vi "FTW-JSON-Interpret-Path.vi"(1 "JSON String":string) -> (0 "LabVIEW Path":path)   [LabVIEW 2015]
panel:
  # "Inputs"
  # "Outputs"
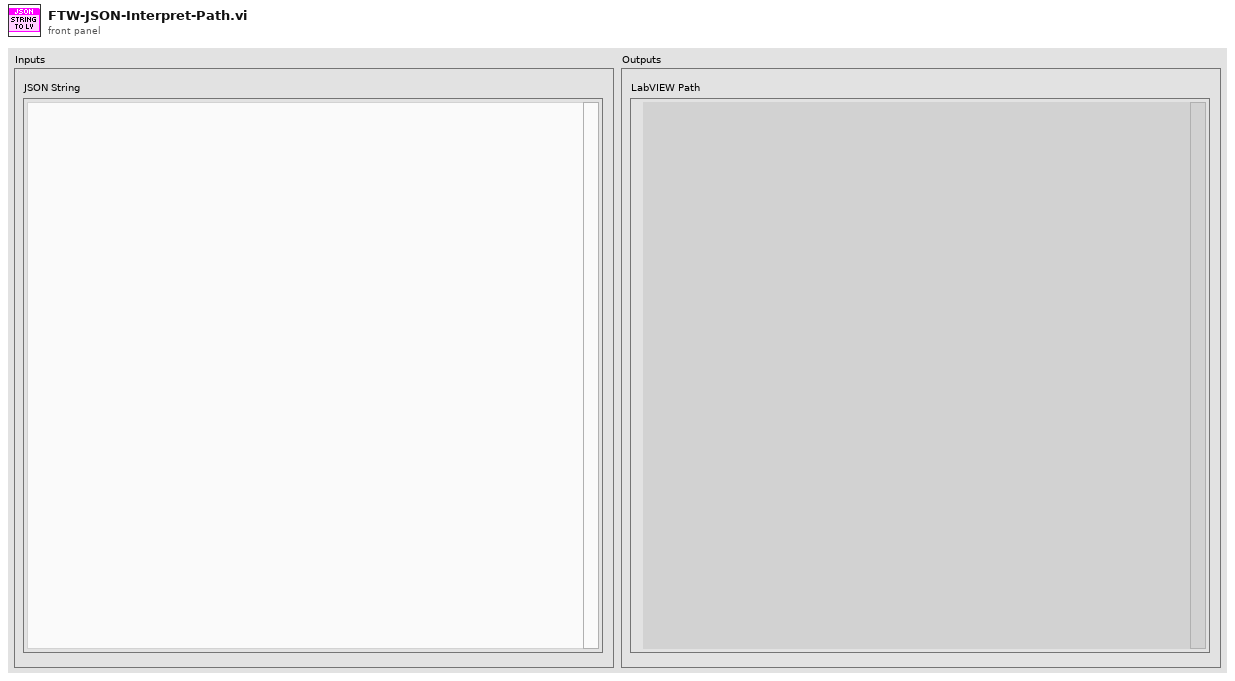
[diagram p1: front panel]
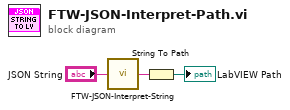
[diagram p0: block diagram]
diagram:
  n1 = call "FTW-JSON-Interpret-String.vi"("JSON String"="JSON String") -> ("LabVIEW String"=w2:string)
  n2 = String To Path(string=w2) -> (path=→"LabVIEW Path":path)
